vi "GradientFilter.vi"(0 "Array":dbl[](array[numeric]), 1 "init/cont (init:F)":bool) -> (2 "Decimated Array":dbl[](array[numeric]))   [LabVIEW 2014]
uses:
  <vilib>/Analysis/3filter.llb/Filter Passband Type.ctl
  <vilib>/Analysis/3filter.llb/Butterworth Filter (DBL).vi
  <vilib>/Analysis/NI_AALBase.lvlib
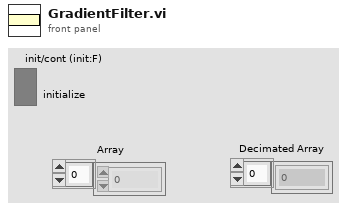
[diagram p1: front panel]
types:
  T1 = typedef "NI_AALBase.lvlib/Filter Passband Type.ctl" = enum32{"Lowpass", "Highpass", "Bandpass", "Bandstop"}
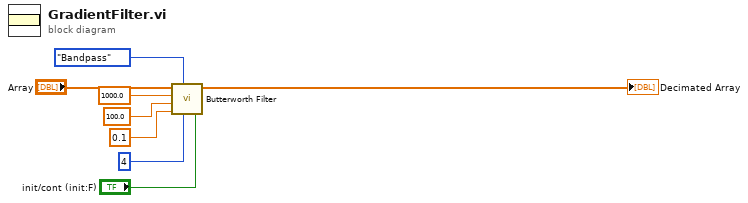
[diagram p0: block diagram]
diagram:
  n1 = call-poly <vilib>:"Butterworth Filter.vi"("init/cont (init:F)"="init/cont (init:F)", "order"=4, "filter type"=Filter_Passband_Type."Bandpass", "low cutoff freq: fl"=0.1, "high cutoff freq: fh"=100.0 ("low cutoff freq: fl"), "sampling freq: fs"=1000.0, "X"="Array") -> ("Filtered X"=→"Decimated Array":dbl[])  [unwired: 1 in, 1 out]
